vi "Y.vi"(8 "error in (no error)":errorcluster, 10 "Wire in":T1, 11 "Gate in":refnum<class "G-UE.lvclass">) -> (0 "error out":errorcluster, 3 "Gate out":refnum<class "G-UE.lvclass">)   [LabVIEW 2016, in "G-UE.lvclass"]
uses:
  G-UE.lvclass
  TypeDefs/Circuit Cluster.ctl
  GateAbst/GateAbst.lvclass
  <vilib>/Analysis/Matrix/Datatypes/ComplexMatrix.ctl
  <vilib>/Analysis/Matrix/NI_Matrix.lvlib
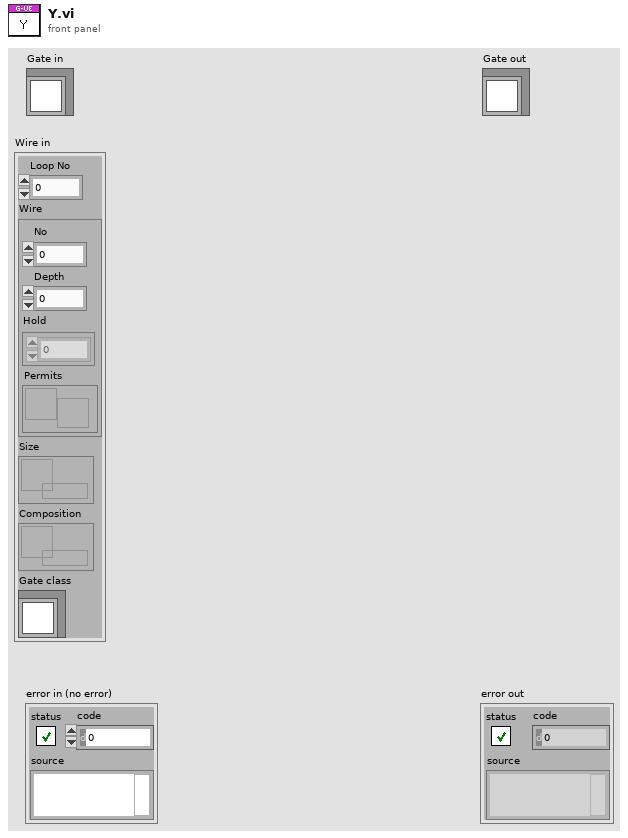
[diagram p1: front panel]
types:
  T1 = typedef "Circuit Cluster.ctl" = cluster{"Loop No":i32, "Wire":cluster{"No":i32, "Depth":i32, "Hold":i32[][], "Permits":refnum<notifier>}, "Size":refnum<queue>, "Composition":refnum<queue>, "Gate class":refnum<class "GateAbst.lvclass">}
  T2 = typedef "NI_Matrix.lvlib/ComplexMatrix.ctl" = cdb[][]
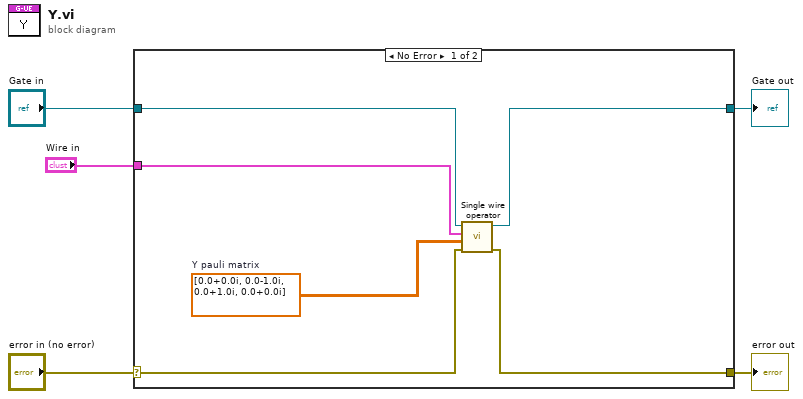
[diagram p0: block diagram]
diagram:
  n1 = case shown="No Error" "error in (no error)" {
    selector: "error in (no error)" -> [w11 w13]
    tunnel: [w7 w13] -> w4
    tunnel: [w9 w12] -> w2
    tunnel: "Gate in" -> [w8 w12]
    tunnel: "Wire in" -> [w6 _]
    frame No Error {
      w10 = T2 [[0.0+0.0i, 0.0-1.0i], [0.0+1.0i, 0.0+0.0i]]  # Y pauli matrix
      n2 = call "Single wire operator.vi"("error in (no error)"=w11, "Operator matrix"=w10, "Wire in"=w6, "G-UE in"=w8) -> ("error out"=w7:errorcluster, "G-UE out"=w9:refnum<class "G-UE.lvclass">)  [unwired: 6 in]
    }
    frame Error {
    }
  }
  "error out" <- w4
  "Gate out" <- w2
